vi "Exchange Param.vi"(8 "error in":errorcluster, 10 "PAR":dbl[](array[numeric]), 11 "Heaters in":refnum<class "Heater.lvclass">[](array[class])) -> (0 "error out":errorcluster, 3 "Heaters out":refnum<class "Heater.lvclass">[](array[class]))   [LabVIEW 2019, in "Heating.lvlib" / "Heater.lvclass"]
uses:
  Heater.lvclass
  Heater.lvclass/Heater.ctl
  HE_state.lvclass/HE_state.ctl
  Z_state/HE_Z_state.lvclass/HE_Z_state.ctl
  ZM_state/HE_ZM_state.lvclass/HE_ZM_state.ctl
  Reg/PID/PID Output Rate Limiter/PID Output Rate Limiter.lvclass
  Reg/PID/PID_OL_AM/PID_OL_AM.lvclass
  D:/my_projects/projects/Algorithms/Labview/19/Reg/PID/PID Output Rate Limiter/PID Output Rate Limiter.lvclass
  Reg/PID/PID_OL_AM/PID_OL_AM.lvclass/PID_OL_AM.ctl
  Reg/PID/PID Output Rate Limiter/PID Output Rate Limiter.lvclass/PID Output Rate Limiter.ctl
  REG/HE_reg.lvclass/HE_reg.ctl
  Reg/PID/PID SP Limiter/PID SP Limiter.lvclass/PID SP Limiter.ctl
  Transform/Impulsator.lvclass/Impulsator.ctl
  REG/HE_reg.lvclass
  D:/my_projects/projects/Algorithms/Labview/19/Reg/PID/PID_OL_AM/PID_OL_AM.lvclass
  Z_state/HE_Z_state.lvclass
  ZM_state/HE_ZM_state.lvclass
  Reg/PID/PID SP Limiter/PID SP Limiter.lvclass
  Transform/Impulsator.lvclass
  HE_state.lvclass
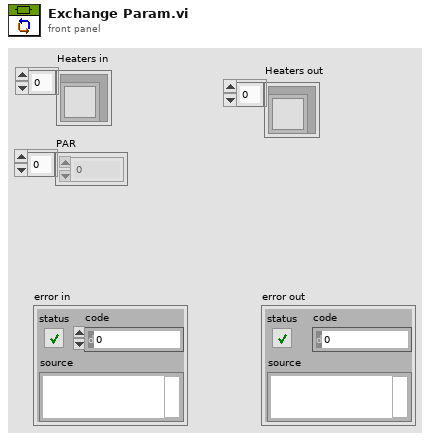
[diagram p1: front panel]
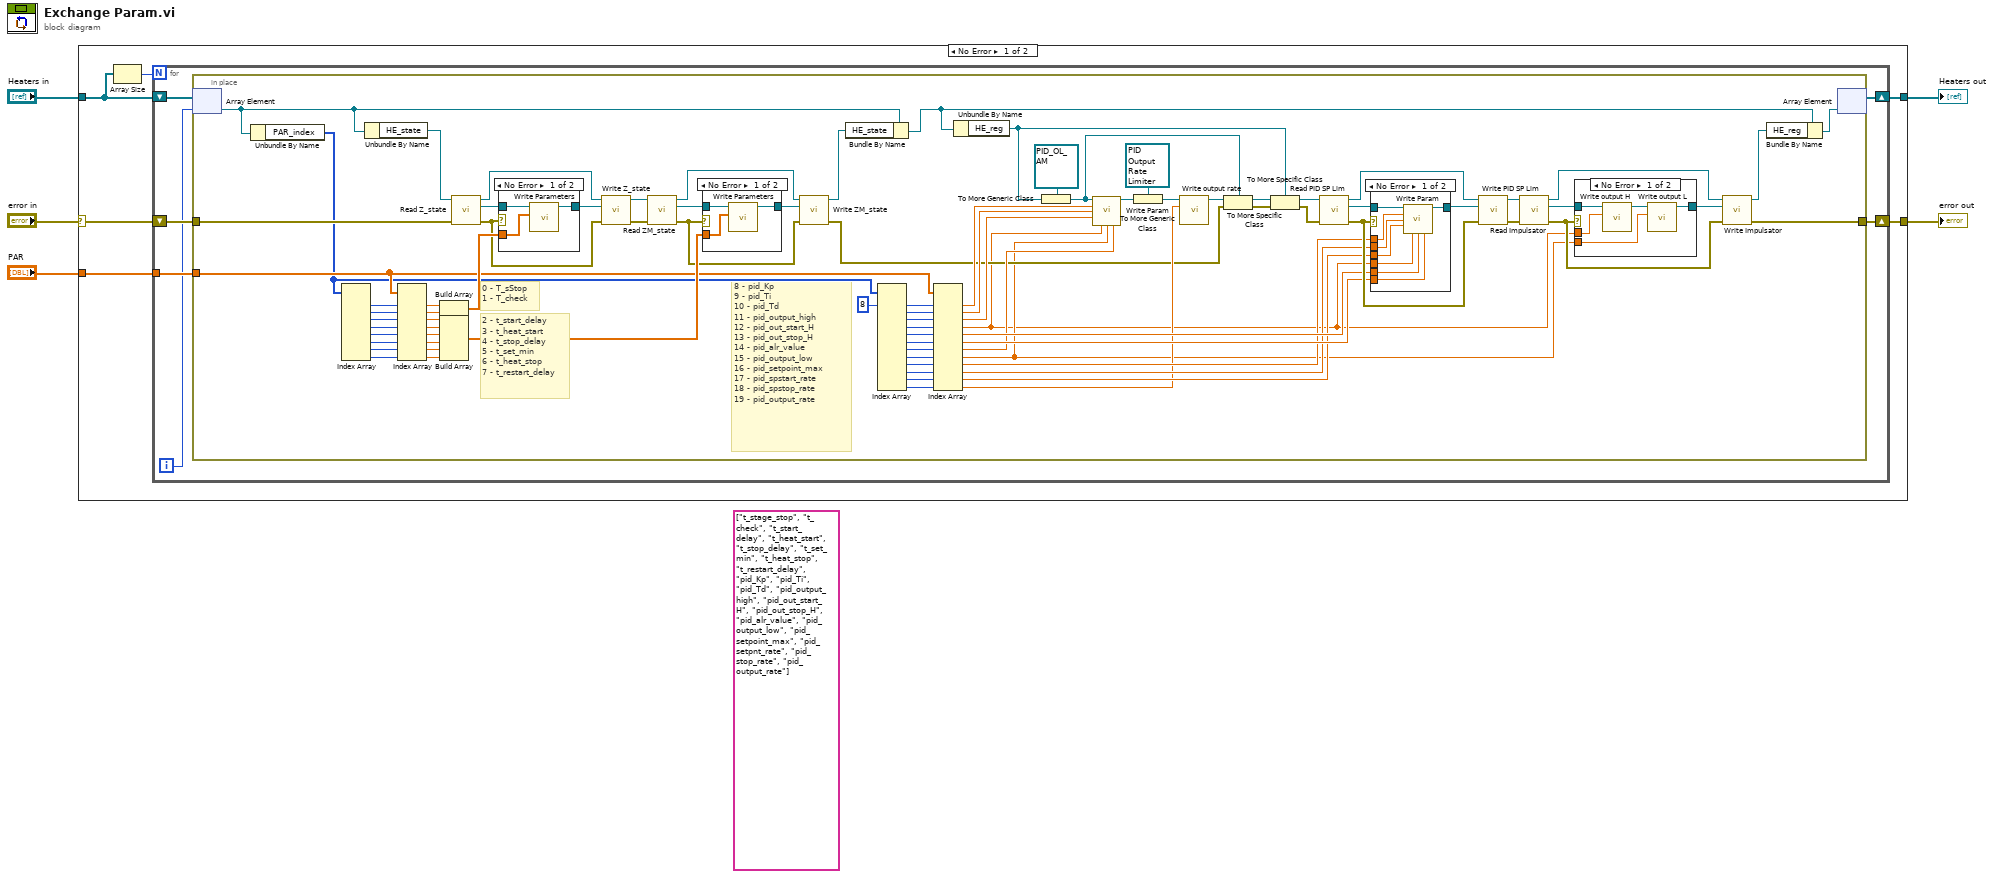
[diagram p0: block diagram]
diagram:
  (unwired) string[] ["t_stage_stop", "t_check", "t_start_delay", "t_heat_start", "t_stop_delay", "t_set_min", "t_heat_stop", "t_restart_delay", "pid_Kp", "pid_Ti", "pid_Td", "pid_output_high", "pid_out_start_H", "pid_out_stop_H", "pid_alr_value", "pid_output_low", "pid_setpoint_max", "pid_setpnt_rate", "pid_stop_rate", "pid_output_rate"]
  n1 = case shown="No Error" "error in" {
    selector: "error in" -> [w8 w126]
    tunnel: [w11 w127] -> w1
    tunnel: "Heaters in" -> [w6 w127]
    tunnel: "PAR" -> [w10 _]
    tunnel: [w9 w126] -> w5
    frame No Error {
      n2 = Array Size(array=w6) -> (size(s)=w7:i32)
      n3 = for {
        N: w7 -> [_]
        tunnel: w10 -> [w17]
        shift-right: [w12] -> w11
        shift-left: w6 -> [w13]
        shift-right: [w16] -> w9
        shift-left: w8 -> [w15]
        i -> [w14]
        n4 = in-place {
          in-place-border: w17 -> [w53]
          in-place-border: [w22] -> w16
          in-place-border: w15 -> [w81]
          # "8 - pid_Kp\n9 - pid_Ti\n10 - pid_Td\n11 - pid_output_high\n12 - pid_out_start_H\n13 - pid_out_stop_H\n14 - pid_alr_value\n15 - pid_output_low\n16 - pid_setpoint_max\n17 - pid_spstart_rate\n18 - pid_spstop_rate\n19 - pid_output_rate"
          # "2 - t_start_delay\n3 - t_heat_start\n4 - t_stop_delay\n5 - t_set_min\n6 - t_heat_stop\n7 - t_restart_delay"
          # "0 - T_sStop\n1 - T_check"
          n5 = in-place-array #1(w13, w14) -> (w71:refnum<class "Heater.lvclass">)
          n6 = Unbundle By Name(w71) -> ("PAR_index"=w52:i32[])
          n7 = Index Array(array=w52) -> (element #1=w102:i32, element #2=w101:i32, element #3=w100:i32, element #4=w96:i32, element #5=w95:i32, element #6=w94:i32, element #7=w93:i32, element #8=w92:i32)  [unwired: 8 in]
          n8 = Unbundle By Name(w71) -> ("HE_state"=w78:refnum<class "HE_state.lvclass">)
          n9 = Index Array(array=w53, index #1=w102, index #2=w101, index #3=w100, index #4=w96, index #5=w95, index #6=w94, index #7=w93, index #8=w92) -> (element #1=w99:dbl, element #2=w98:dbl, element #3=w91:dbl, element #4=w90:dbl, element #5=w89:dbl, element #6=w88:dbl, element #7=w87:dbl, element #8=w86:dbl)
          n10 = Build Array(w99, w98) -> (w97:dbl[])
          n11 = Build Array(w91, w90, w89, w88, w87, w86) -> (w85:dbl[])
          n12 = call "Read Z_state.vi"("error in (no error)"=w81, "HE_state in"=w78) -> ("error out"=w79:errorcluster, "Heating.lvlib:HE_Z_state.lvclass"=w80:refnum<class "HE_Z_state.lvclass">, "HE_state out"=w77:refnum<class "HE_state.lvclass">)  [unwired: 7 in]
          n13 = case shown="No Error" w79 {
            tunnel: w80 -> [w105 w106]
            tunnel: w97 -> [w104 _]
            tunnel: [w103 w106] -> w84
            frame No Error {
              n14 = call "Write Parameters.vi"("Parameters"=w104, "HE1_Z_state in"=w105) -> ("HE1_Z_state out"=w103:refnum<class "HE_Z_state.lvclass">)  [unwired: 9 in]
            }
            frame Error {
            }
          }
          n15 = call "Write Z_state.vi"("error in (no error)"=w79, "Heating.lvlib:HE_Z_state.lvclass"=w84, "HE_state in"=w77) -> ("error out"=w72:errorcluster, "HE_state out"=w76:refnum<class "HE_state.lvclass">)  [unwired: 7 in]
          n16 = call "Read ZM_state.vi"("error in (no error)"=w72, "HE_state in"=w76) -> ("error out"=w74:errorcluster, "HE_ZM_state"=w73:refnum<class "HE_ZM_state.lvclass">, "HE_state out"=w75:refnum<class "HE_state.lvclass">)  [unwired: 7 in]
          n17 = case shown="No Error" w74 {
            tunnel: w73 -> [w109 w110]
            tunnel: [w108 w110] -> w83
            tunnel: w85 -> [w107 _]
            frame No Error {
              n18 = call "Write Parameters.vi"("Parameters"=w107, "valve_VCH_ZM_state in"=w109) -> ("valve_VCH_ZM_state out"=w108:refnum<class "HE_ZM_state.lvclass">)  [unwired: 9 in]
            }
            frame Error {
            }
          }
          n19 = call "Write ZM_state.vi"("error in (no error)"=w74, "HE_ZM_state"=w83, "HE_state in"=w75) -> ("error out"=w25:errorcluster, "HE_state out"=w82:refnum<class "HE_state.lvclass">)  [unwired: 7 in]
          n20 = Bundle By Name(cluster=w71, "HE_state"=w82) -> (w20:refnum<class "Heater.lvclass">)
          n21 = Index Array(array=w52, index #1=8 ("index")) -> (element #1=w50:i32, element #2=w54:i32, element #3=w55:i32, element #4=w56:i32, element #5=w57:i32, element #6=w58:i32, element #7=w59:i32, element #8=w60:i32, element #9=w49:i32, element #10=w48:i32, element #11=w47:i32, element #12=w46:i32)  [unwired: 11 in]
          n22 = Index Array(array=w53, index #1=w50, index #2=w54, index #3=w55, index #4=w56, index #5=w57, index #6=w58, index #7=w59, index #8=w60, index #9=w49, index #10=w48, index #11=w47, index #12=w46) -> (element #1=w45:dbl, element #2=w44:dbl, element #3=w43:dbl, element #4=w18:dbl, element #5=w42:dbl, element #6=w41:dbl, element #7=w40:dbl, element #8=w23:dbl, element #9=w39:dbl, element #10=w38:dbl, element #11=w37:dbl, element #12=w29:dbl)
          n23 = Unbundle By Name(w20) -> ("HE_reg"=w35:refnum<class "HE_reg.lvclass">)
          n24 = To More Generic Class(target class=refnum<class "PID_OL_AM.lvclass"> refnum ("control.lvlib:PID_OL_AM.lvclass"), reference=w35) -> (generic class reference=w26:refnum<class "PID_OL_AM.lvclass">)
          n25 = call "Write Param.vi"("PID_OL_AM in"=w26, "Kc"=w45, "Ti"=w44, "Td"=w43, "output H"=w18, "output L"=w23, "alr value"=w40) -> ("PID_OL_AM out"=w32:refnum<class "PID_OL_AM.lvclass">)  [unwired: 8 in]
          n26 = To More Generic Class(target class=refnum<class "PID Output Rate Limiter.lvclass"> refnum ("control.lvlib:PID Output Rate Limiter.lvclass"), reference=w32) -> (generic class reference=w30:refnum<class "PID Output Rate Limiter.lvclass">)
          n27 = call "Write output rate.vi"("output rate"=w29, "PID Output Rate Limiter in"=w30) -> ("PID Output Rate Limiter out"=w27:refnum<class "PID Output Rate Limiter.lvclass">)  [unwired: 9 in]
          n28 = To More Specific Class(target class=w26, reference=w27, error in=w25) -> (specific class reference=w28:refnum<class "PID_OL_AM.lvclass">, error out=w24:errorcluster)
          n29 = To More Specific Class(target class=w35, reference=w28, error in=w24) -> (specific class reference=w33:refnum<class "HE_reg.lvclass">, error out=w34:errorcluster)
          n30 = call "Read PID SP Lim.vi"("error in (no error)"=w34, "HE_reg in"=w33) -> ("error out"=w68:errorcluster, "PID SP Limiter"=w70:refnum<class "PID SP Limiter.lvclass">, "HE_reg out"=w69:refnum<class "HE_reg.lvclass">)  [unwired: 7 in]
          n31 = case shown="No Error" w68 {
            tunnel: w70 -> [w118 w119]
            tunnel: [w117 w119] -> w62
            tunnel: w39 -> [w116 _]
            tunnel: w38 -> [w115 _]
            tunnel: w37 -> [w114 _]
            tunnel: w42 -> [w112 _]
            tunnel: w41 -> [w111 _]
            tunnel: w18 -> [w113 _]
            frame No Error {
              n32 = call "Write Param.vi"("PID SP Limiter in"=w118, "SP_max"=w116, "SP_start_rate"=w115, "SP_stop_rate"=w114, "Out_H"=w113, "Out_start_H"=w112, "Out_stop_H"=w111) -> ("PID SP Limiter out"=w117:refnum<class "PID SP Limiter.lvclass">)  [unwired: 8 in]
            }
            frame Error {
            }
          }
          n33 = call "Write PID SP Lim.vi"("error in (no error)"=w68, "PID SP Limiter"=w62, "HE_reg in"=w69) -> ("error out"=w66:errorcluster, "HE_reg out"=w67:refnum<class "HE_reg.lvclass">)  [unwired: 7 in]
          n34 = call "Read Impulsator.vi"("error in (no error)"=w66, "HE_reg in"=w67) -> ("error out"=w63:errorcluster, "Impulsator"=w65:refnum<class "Impulsator.lvclass">, "HE_reg out"=w64:refnum<class "HE_reg.lvclass">)  [unwired: 7 in]
          n35 = case shown="No Error" w63 {
            tunnel: w65 -> [w124 w125]
            tunnel: [w122 w125] -> w61
            tunnel: w18 -> [w121 _]
            tunnel: w23 -> [w120 _]
            frame No Error {
              n36 = call "Write output H.vi"("output H"=w121, "Impulsator in"=w124) -> ("Impulsator out"=w123:refnum<class "Impulsator.lvclass">)  [unwired: 9 in]
              n37 = call "Write output L.vi"("output L"=w120, "Impulsator in"=w123) -> ("Impulsator out"=w122:refnum<class "Impulsator.lvclass">)  [unwired: 9 in]
            }
            frame Error {
            }
          }
          n38 = call "Write Impulsator.vi"("error in (no error)"=w63, "Impulsator"=w61, "HE_reg in"=w64) -> ("error out"=w22:errorcluster, "HE_reg out"=w21:refnum<class "HE_reg.lvclass">)  [unwired: 7 in]
          n39 = Bundle By Name(cluster=w20, "HE_reg"=w21) -> (w19:refnum<class "Heater.lvclass">)
          n40 = in-place-array #1(w19) -> (w12:refnum<class "Heater.lvclass">[])  [unwired: 1 out]
        }
      }
    }
    frame Error {
    }
  }
  "error out" <- w5
  "Heaters out" <- w1
